vi "FRCts20_Backend_RequestRoot_GET_reform.vi"(7 "Request Root":T1, 8 "error in (no error)":errorcluster, 11 "recordset data":variant[][](array[variant])) -> (0 "error out":errorcluster, 3 "data string":string)   [LabVIEW 2013, in "FRCts20_Backend_Engine.lvlib"]
doc: "Reforms and returns the list of requests' data"
uses:
  FRCts20_Backend_Engine.lvlib
  FRCts20_Backend_API/FRCts20_Backend_API_RequestRoot.ctl
  FRCts20_Backend_API/FRCts20_Backend_API_Status.ctl
  FRCts20_Backend_DBCluster_RequestRoot_GET.ctl
  <vilib>/addons/database/_DB Variant To Data/Database Variant To Data.xnode
  FRCts20_Backend_API/FRCts20_Backend_API.lvlib
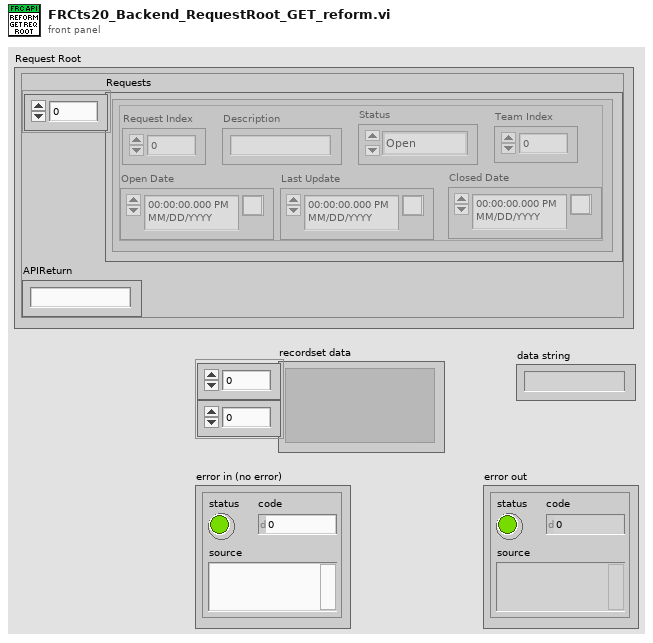
[diagram p1: front panel]
types:
  T1 = typedef "FRCts20_Backend_API.lvlib/FRCts20_Backend_API_RequestRoot.ctl" = cluster{"Requests":cluster{"Request Index":u32, "Description":string, "Status":T2, "Open Date":timestamp, "Last Update":timestamp, "Closed Date":timestamp, "Team Index":u32}[], "APIReturn":string}
  T2 = typedef "FRCts20_Backend_API.lvlib/FRCts20_Backend_API_Status.ctl" = enum16{"Open", "In Work", "Closed"}
  T3 = typedef "FRCts20_Backend_Engine.lvlib/FRCts20_Backend_DBCluster_RequestRoot_GET.ctl" = cluster{"ReqNumber":u32, "TeamIndex":u32, "Description":string, "Status":u16, "OpenDate":timestamp, "LastUpdate":timestamp, "CloseDate":timestamp}
  T4 = cluster{"Request Index":u32, "Description":string, "Status":T2, "Open Date":timestamp, "Last Update":timestamp, "Closed Date":timestamp, "Team Index":u32}[]
  T5 = cluster{"Request Index":u32, "Description":string, "Status":T2, "Open Date":timestamp, "Last Update":timestamp, "Closed Date":timestamp, "Team Index":u32}
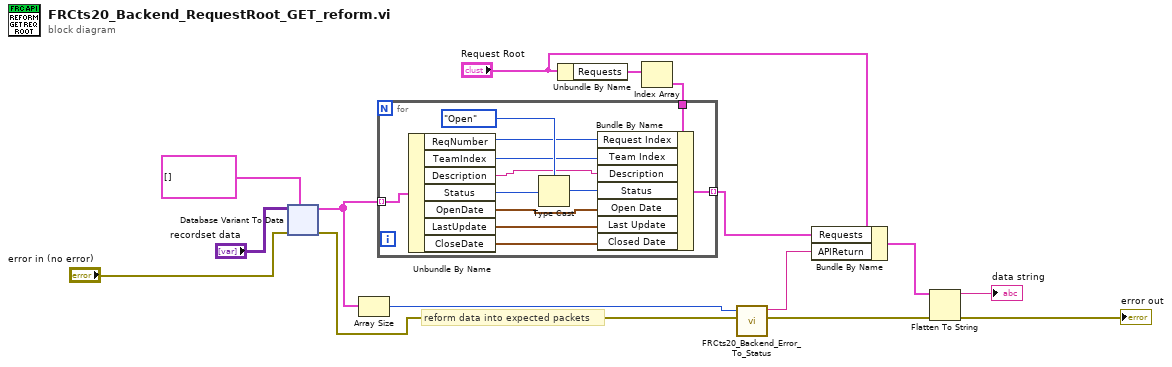
[diagram p0: block diagram]
diagram:
  # "reform data into expected packets"
  n1 = xnode "Database Variant To Data"("database variant"="recordset data", "error in (no error)"="error in (no error)", "type"=T3[] []) -> ("data"=w3:T3[], "error out"=w10:errorcluster)
  n2 = Array Size(array=w3) -> (size(s)=w11:i32)
  n3 = Unbundle By Name("Request Root") -> ("Requests"=w4:T4)
  n4 = Index Array(array=w4) -> (element=w5:T5)  [unwired: 1 in]
  n5 = for {
    tunnel: [w20] -> w1 mode=indexing
    tunnel: w5 -> [w18]
    tunnel: w3 -> [w17] mode=indexing
    n6 = Unbundle By Name(w17) -> ("ReqNumber"=w16:u32, "TeamIndex"=w25:u32, "Description"=w24:string, "Status"=w27:u16, "OpenDate"=w22:timestamp, "LastUpdate"=w21:timestamp, "CloseDate"=w19:timestamp)
    n7 = Type Cast(type=FRCts20_Backend_API_Status."Open" ("Status"), x=w27) -> (*(type *) &x=w23:T2)
    n8 = Bundle By Name(cluster=w18, "Request Index"=w16, "Team Index"=w25, "Description"=w24, "Status"=w23, "Open Date"=w22, "Last Update"=w21, "Closed Date"=w19) -> (w20:T5)
  }
  n9 = call "FRCts20_Backend_Error_To_Status.vi"("error in (no error)"=w10, "rows affected"=w11) -> ("error out"=w12:errorcluster, "String"=w13:string)  [unwired: 8 in]
  n10 = Bundle By Name(cluster="Request Root", "Requests"=w1, "APIReturn"=w13) -> (w8:T1)
  n11 = Flatten To String(anything=w8, error in (no error)=w12) -> (data string=→"data string":string, error out=→"error out":errorcluster)  [unwired: 2 in, 1 out]
